vi "name2ref.vi"(3 "error in (no error)":errorcluster, 5 "name":string) -> (0 "error out":errorcluster, 1 "obj exists":bool, 2 "objectRef out":refnum<class "HGF_Reference.lvclass">)   [LabVIEW 2012, in "HGF_ObjectManager.lvlib"]
doc: "This VI returns the reference of the named object."
uses:
  HGF_ObjectManager.lvlib
  HGF_BaseClasses/HGF_Reference/HGF_Reference.lvclass
  action.ctl
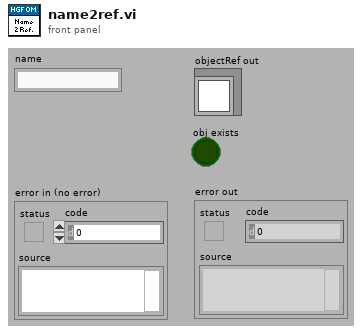
[diagram p1: front panel]
types:
  T1 = typedef "HGF_ObjectManager.lvlib/action.ctl" = enum16{"add", "remove", "name2ref", "ref2name ", "obj exists?", "cleanup", "get object list", "reset"}
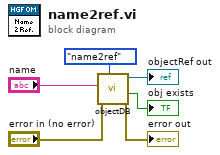
[diagram p0: block diagram]
diagram:
  n1 = call "objectDB.vi"("Action"=action."name2ref", "error in (no error)"="error in (no error)", "name"="name") -> ("error out"=→"error out":errorcluster, "obj exists"=→"obj exists":bool, "objectRef out"=→"objectRef out":refnum<class "HGF_Reference.lvclass">)  [unwired: 2 in, 4 out]
